vi "testShould Count The Number Of Calls.vi"(8 "error in (no error)":errorcluster, 11 "TestCase in":refnum<class "RegisterCalls.lvclass">) -> (0 "error out":errorcluster, 3 "TestCase out":refnum<class "RegisterCalls.lvclass">)   [LabVIEW 2013, in "RegisterCalls.lvclass"]
uses:
  RegisterCalls.lvclass
  Core Classes/LabSpy/LabSpy.lvclass
  <vilib>/addons/_JKI Toolkits/VI Tester/TestCase.llb/TestCase.lvclass
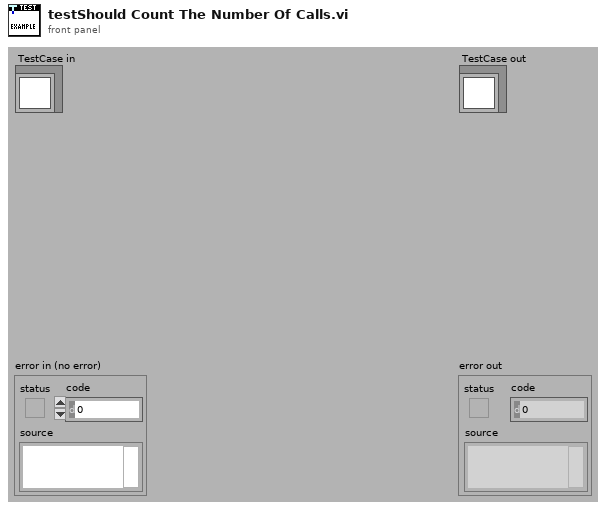
[diagram p1: front panel]
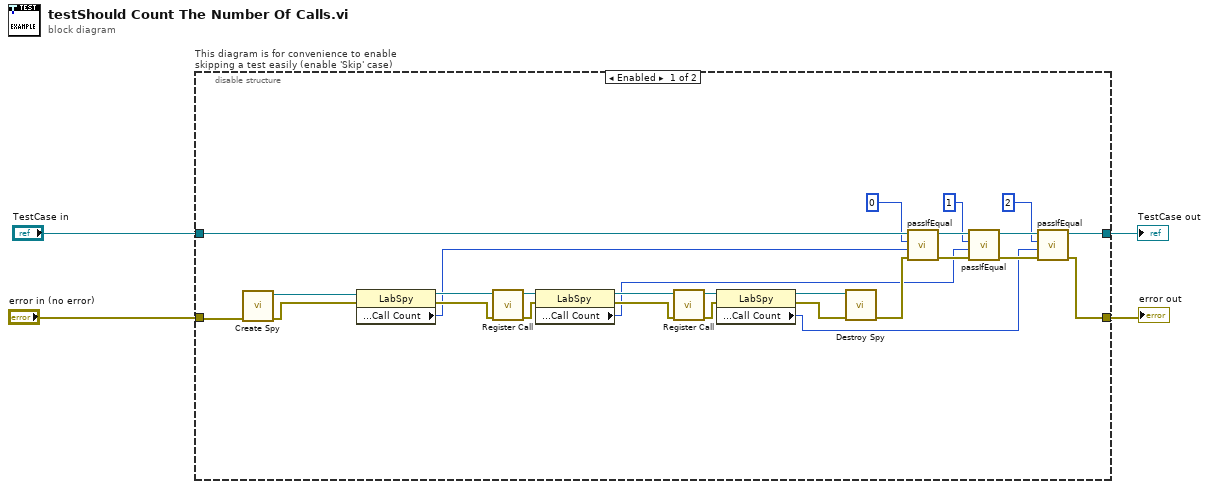
[diagram p0: block diagram]
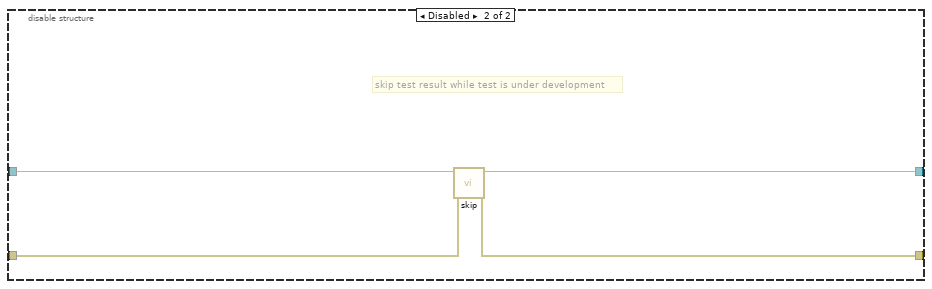
[diagram p2: hidden frame]
diagram:
  n1 = disable-structure "This diagram is for convenience to enable skipping a test easily (enable 'Skip' case)" shown="Enabled" {
    disable-tunnel: "TestCase in" -> [w15 w35]
    disable-tunnel: [w18 w33] -> w1
    disable-tunnel: [w11 w34] -> w3
    disable-tunnel: "error in (no error)" -> [w31 w32]
    frame Enabled {
      n2 = call "Create Spy.vi"("error in (no error)"=w31) -> ("error out"=w30:errorcluster, "LabSpy Out"=w29:refnum<data-value>)  [unwired: 9 in]
      n3 = property class="LabSpy"(reference=w29, error in=w30) -> (reference out=w26:refnum<data-value>, error out=w25:errorcluster, "Call Monitoring:Call Count"=w8:i32)
      n4 = call "Register Call.vi"("error in (no error)"=w25, "LabSpy"=w26) -> ("error out"=w28:errorcluster, "LabSpy Out"=w27:refnum<data-value>)  [unwired: 8 in]
      n5 = property class="LabSpy"(reference=w27, error in=w28) -> (reference out=w22:refnum<data-value>, error out=w21:errorcluster, "Call Monitoring:Call Count"=w9:i32)
      n6 = call "Register Call.vi"("error in (no error)"=w21, "LabSpy"=w22) -> ("error out"=w24:errorcluster, "LabSpy Out"=w23:refnum<data-value>)  [unwired: 8 in]
      n7 = property class="LabSpy"(reference=w23, error in=w24) -> (reference out=w20:refnum<data-value>, error out=w19:errorcluster, "Call Monitoring:Call Count"=w10:i32)
      n8 = call "Destroy Spy.vi"("error in (no error)"=w19, "LabSpy"=w20) -> ("error out"=w14:errorcluster)  [unwired: 9 in]
      n9 = call-dynamic "passIfEqual.vi"("error in (no error)"=w14, "y"=w8, "x"=0 ("Call Count"), "TestCase in"=w15) -> ("error out"=w13:errorcluster, "TestCase out"=w16:refnum<class "RegisterCalls.lvclass">)  [unwired: 6 in]
      n10 = call-dynamic "passIfEqual.vi"("error in (no error)"=w13, "y"=w9, "x"=1 ("Call Count"), "TestCase in"=w16) -> ("error out"=w12:errorcluster, "TestCase out"=w17:refnum<class "RegisterCalls.lvclass">)  [unwired: 6 in]
      n11 = call-dynamic "passIfEqual.vi"("error in (no error)"=w12, "y"=w10, "x"=2 ("Call Count"), "TestCase in"=w17) -> ("error out"=w11:errorcluster, "TestCase out"=w18:refnum<class "RegisterCalls.lvclass">)  [unwired: 6 in]
    }
    frame Disabled {
      # "skip test result while test is under development"
      n12 = call <vilib>:"skip.vi"("error in (no error)"=w32, "TestCase in"=w35) -> ("error out"=w34:errorcluster, "TestCase out"=w33:refnum<class "RegisterCalls.lvclass">)  [unwired: 8 in]
    }
  }
  "error out" <- w3
  "TestCase out" <- w1
